vi "StartAutoTest.vi"(8 "error in (no error)":errorcluster, 11 "ExecutionControls in":refnum<class "ExecutionControls.lvclass">) -> (0 "error out":errorcluster, 3 "ExecutionControls out":refnum<class "ExecutionControls.lvclass">)   [LabVIEW 2018, in "ExecutionControls.lvclass"]
uses:
  ExecutionControls.lvclass
  <vilib>/Utility/miscctls.llb/LVForegroundBackgroundColorsTypeDef.ctl
  ExecutionControls.lvclass/ExecutionControls.ctl
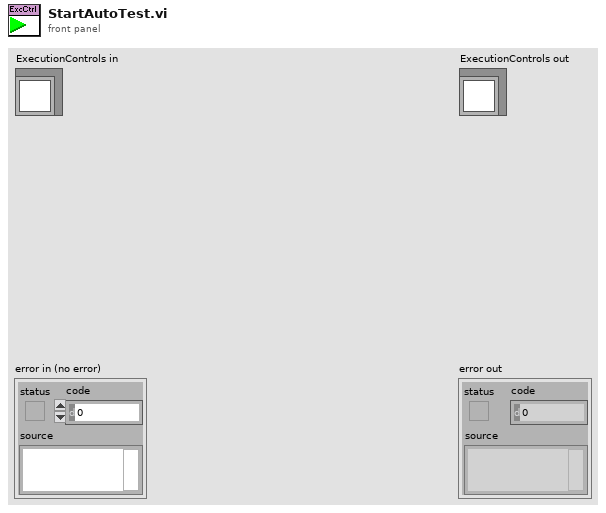
[diagram p1: front panel]
types:
  T1 = enum32{"Page Enabled", "Page Disabled", "Page Disabled & Grayed"}
  T2 = enum8{"Enabled", "Disabled", "Disabled and Grayed Out"}
  T3 = typedef "LVForegroundBackgroundColorsTypeDef.ctl" = cluster{"Foreground Color":u32, "Background Color":u32}
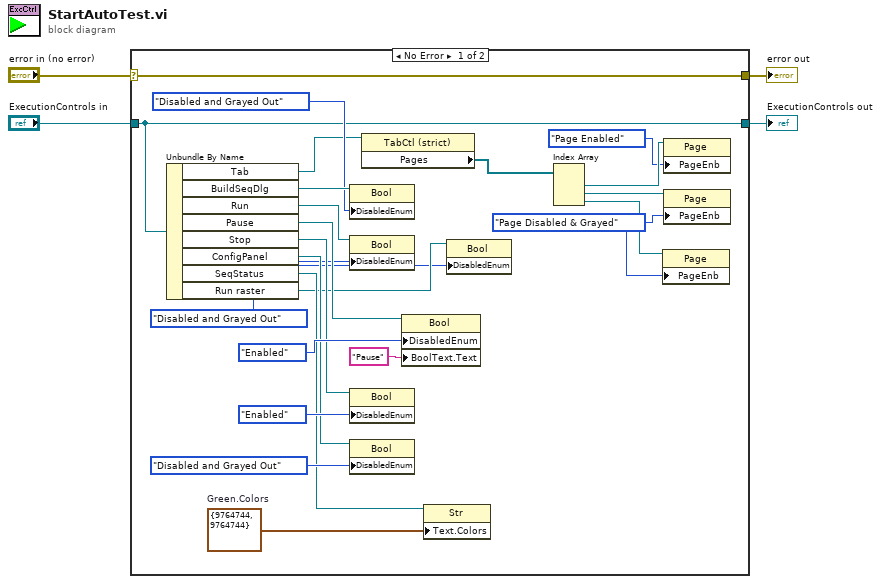
[diagram p0: block diagram]
diagram:
  n1 = case shown="No Error" "error in (no error)" {
    selector: "error in (no error)" -> [w27 w29]
    tunnel: [w27 w29] -> w3
    tunnel: [w17 w28] -> w1
    tunnel: "ExecutionControls in" -> [w17 w28]
    frame No Error {
      w9 = T3 {"Foreground Color"=9764744, "Background Color"=9764744}  # Green.Colors
      w7 = T1."Page Disabled & Grayed" ("Page Enabled State")
      w5 = T2."Disabled and Grayed Out" ("Disabled")
      n2 = Unbundle By Name(w17) -> ("Tab"=w16:refnum<vi>, "BuildSeqDlg"=w26:refnum<vi>, "Run"=w24:refnum<vi>, "Pause"=w20:refnum<vi>, "Stop"=w19:refnum<vi>, "ConfigPanel"=w18:refnum<vi>, "SeqStatus"=w10:refnum<vi>, "Run raster"=w6:refnum<vi>)
      n3 = property class="Bool"(reference=w26, "DisabledEnum"=T2."Disabled and Grayed Out" ("Disabled")) -> ()  [unwired: 1 in, 2 out]
      n4 = property class="Bool"(reference=w24, "DisabledEnum"=w5) -> ()  [unwired: 1 in, 2 out]
      n5 = property class="Bool"(reference=w19, "DisabledEnum"=T2."Enabled" ("Disabled")) -> ()  [unwired: 1 in, 2 out]
      n6 = property class="Bool"(reference=w18, "DisabledEnum"=T2."Disabled and Grayed Out" ("Disabled")) -> ()  [unwired: 1 in, 2 out]
      n7 = property class="TabCtl (strict)"(reference=w16) -> ("Pages"=w15:refnum<vi>[])  [unwired: 1 in, 2 out]
      n8 = property class="Bool"(reference=w20, "DisabledEnum"=T2."Enabled" ("Disabled"), "BoolText.Text"="Pause" ("Boolean Text.Text")) -> ()  [unwired: 1 in, 2 out]
      n9 = property class="Str"(reference=w10, "Text.Colors"=w9) -> ()  [unwired: 1 in, 2 out]
      n10 = property class="Bool"(reference=w6, "DisabledEnum"=w5) -> ()  [unwired: 1 in, 2 out]
      n11 = Index Array(array=w15) -> (element #1=w13:refnum<vi>, element #2=w14:refnum<vi>, element #3=w8:refnum<vi>)  [unwired: 3 in]
      n12 = property class="Page"(reference=w8, "PageEnb"=w7) -> ()  [unwired: 1 in, 2 out]
      n13 = property class="Page"(reference=w13, "PageEnb"=T1."Page Enabled" ("Page Enabled State")) -> ()  [unwired: 1 in, 2 out]
      n14 = property class="Page"(reference=w14, "PageEnb"=w7) -> ()  [unwired: 1 in, 2 out]
    }
    frame Error {
    }
  }
  "error out" <- w3
  "ExecutionControls out" <- w1
